vi "IT7800 Close.vi"(8 "error in":errorcluster, 11 "VISA in":refnum<visa-resource-name>="TCPIP::192.168.0.252") -> (0 "error out":errorcluster, 3 "VISA out":refnum<visa-resource-name>)   [LabVIEW 2025]
uses:
  <instrlib>/IT7800/IT7800.lvlib
panel:
  # "IP7800 Driver V0.10\nClose"
  # "06.05.2025"
  # "Andrej Valand"
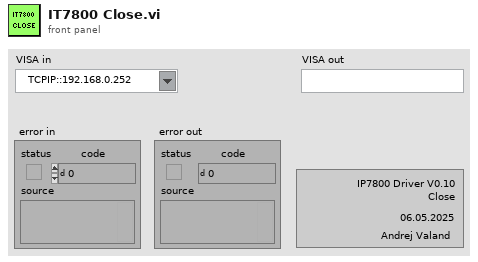
[diagram p1: front panel]
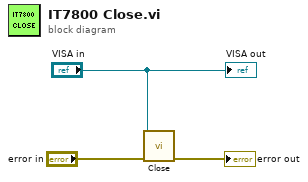
[diagram p0: block diagram]
diagram:
  n1 = call <instrlib>:"Close.vi"("error in"="error in", "VISA resource name"="VISA in") -> ("error out"=→"error out":errorcluster)  [unwired: 9 in]
  "VISA out" <- "VISA in"
